vi "stop_A.vi"() -> ()   [LabVIEW 2013]
panel:
  in  "stop_A":bool
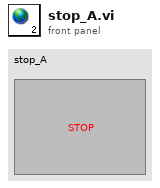
[diagram p1: front panel]
diagram:
